vi "onSuiteSlippage.vi"(7 "DefineSuite in":refnum<class "DefineSuite.lvclass">, 11 "Leaf.TestSuite":refnum<class "Leaf.TestSuite.lvclass">) -> (0 "error out":errorcluster, 3 "Leaf.TestSuite":refnum<class "Leaf.TestSuite.lvclass">)   [LabVIEW 2021, in "Bananas.lvlib" / "DefineSuite.lvclass"]
uses:
  DefineSuite.lvclass
  Leaf.TestSuite/Leaf.TestSuite.lvclass
  DefineSuite.lvclass/DefineSuite.ctl
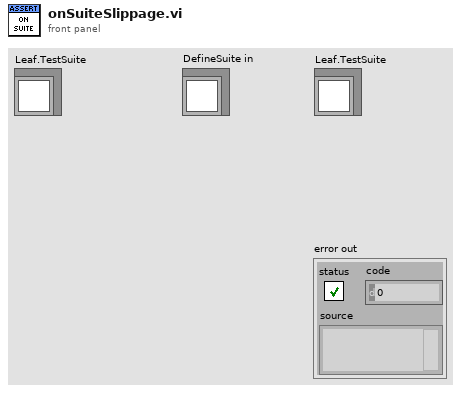
[diagram p1: front panel]
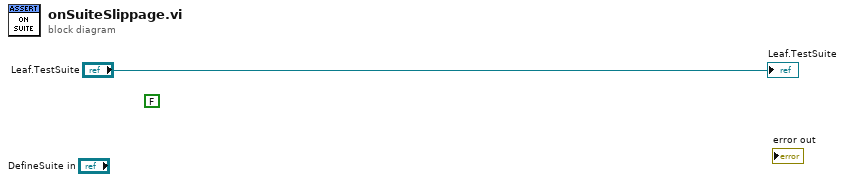
[diagram p0: block diagram]
diagram:
  (unwired) FALSE
  "Leaf.TestSuite" <- "Leaf.TestSuite"
